vi "Config Puerto.vi"(11 "Data Cluster":T1={"VISA resource name"="ASRL4::INSTR"}) -> (3 "Data Cluster Out":T1={"VISA resource name"="ASRL4::INSTR"})   [LabVIEW 2020, in "Serial Device.lvclass"]
uses:
  Serial Device.lvclass
  Data Cluster.ctl
panel:
  in  "OK Button":bool
  in  "VISA resource name":refnum<visa-resource-name>="ASRL4::INSTR"
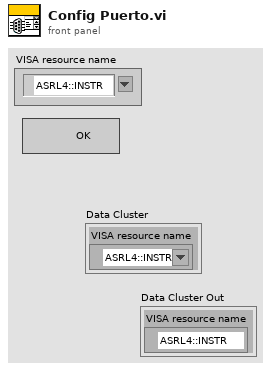
[diagram p1: front panel]
types:
  T1 = typedef "Data Cluster.ctl" = cluster{"VISA resource name":refnum<visa-resource-name>}
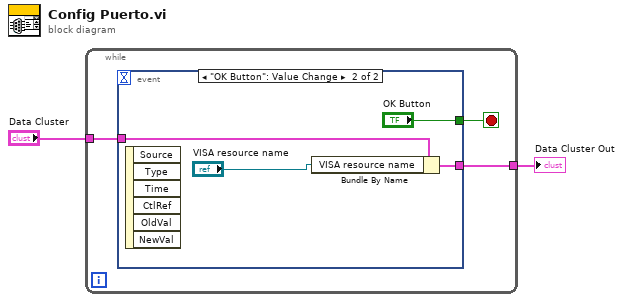
[diagram p0: block diagram]
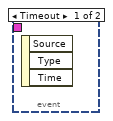
[diagram p2: hidden frame]
diagram:
  n1 = while {
    tunnel: "Data Cluster" -> [w5]
    tunnel: [w4] -> w1
    stop <- w3 stop-if-true
    n2 = event shown="[1] \"OK Button\": Value Change" {
      selector: _ -> [_ _]
      dyn-events: _ -> [_ _]
      timeout: _ -> [_ _]
      tunnel: w5 -> [_ w9]
      tunnel: [_ w8] -> w4
      tunnel: [_ "OK Button"] -> w3
      event Timeout {
        n3 = event-data() -> ()  [unwired: 1 in, 3 out]
      }
      event "OK Button": Value Change {
        n4 = event-data() -> ()  [unwired: 1 in, 6 out]
        n5 = Bundle By Name(cluster=w9, "VISA resource name"="VISA resource name") -> (w8:T1)
      }
    }
  }
  "Data Cluster Out" <- w1
